vi "PC_testbench_for_FPGA_VI.vi"() -> ()   [LabVIEW 2020]
uses:
  <vilib>/rvi/DesktopExecutionNode/Execution/niFpgaDEN_Execute.vi
  <vilib>/rvi/DesktopExecutionNode/DesktopExecutionNode.xnode
panel:
  in  "Reset Photon Count":bool
  in  "Type Counter":enum16{"Falling Edge", "Rising Edge"}(ring)
  out "Mod2/DIO0 2":bool
  in  "SPCM Pulse":bool
  out "Photon Counts 1":i32
  in  "Stop execution":bool
  # "FPGA VI Test Bench"
  # "FPGA VI Inputs"
  # "FPGA VI Outputs"
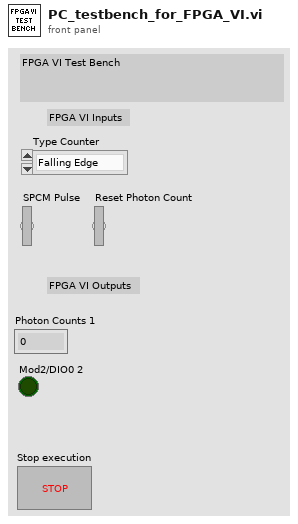
[diagram p1: front panel]
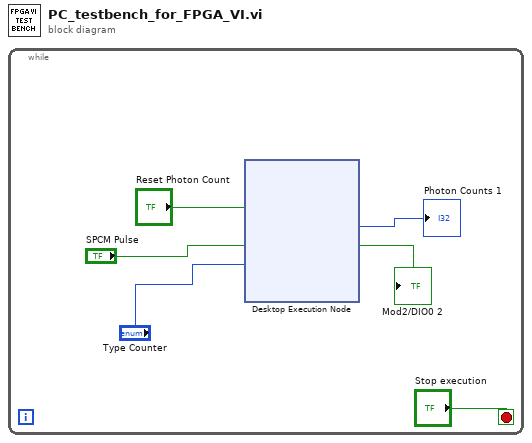
[diagram p0: block diagram]
diagram:
  n1 = while {
    stop <- "Stop execution" stop-if-true
    n2 = xnode "Desktop Execution Node"("Mod2/DIO0"="SPCM Pulse", "Type Counter"="Type Counter", "Reset Photon Count"="Reset Photon Count") -> ("Total Counts"=→"Photon Counts 1":i32, "Mod2/DIO0"=→"Mod2/DIO0 2":bool)  [unwired: 1 in, 1 out]
  }
